vi "oa_TV Average Angle Intervals (1Chan).vi"(6 "revulotion index":i32, 7 "reset? (F)":bool, 8 "error in (no error)":errorcluster, 9 "pulse/revolution":i32, 10 "RPM":dbl[](array[numeric]), 11 "time index":dbl[](array[numeric]) format="%.2f") -> (0 "error out":errorcluster, 3 "angle intervals":dbl[](array[numeric]))   [LabVIEW 2017, in "SoundVib_Torsional.lvlib"]
uses:
  <vilib>/addons/Sound and Vibration/Order Analysis/Torsional Vibration/SoundVib_Torsional.lvlib
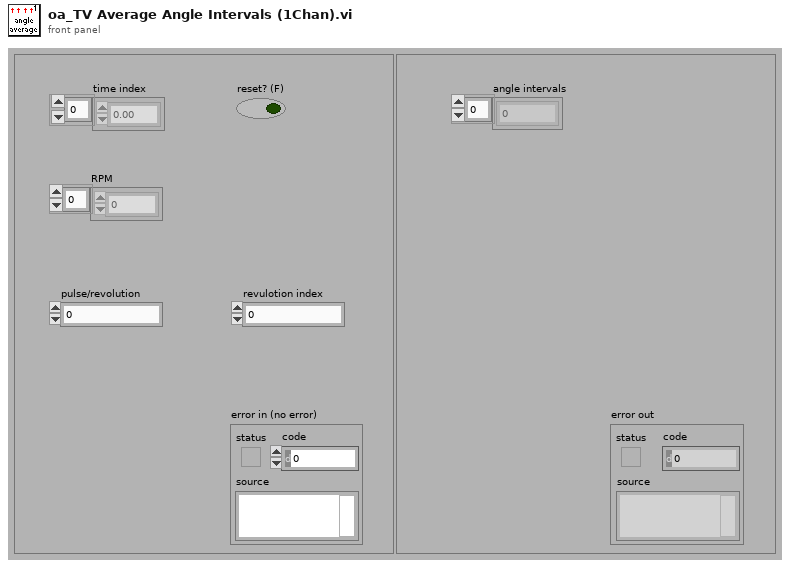
[diagram p1: front panel]
types:
  T1 = enum16{"Exponential average", "Moving average", "Current"}
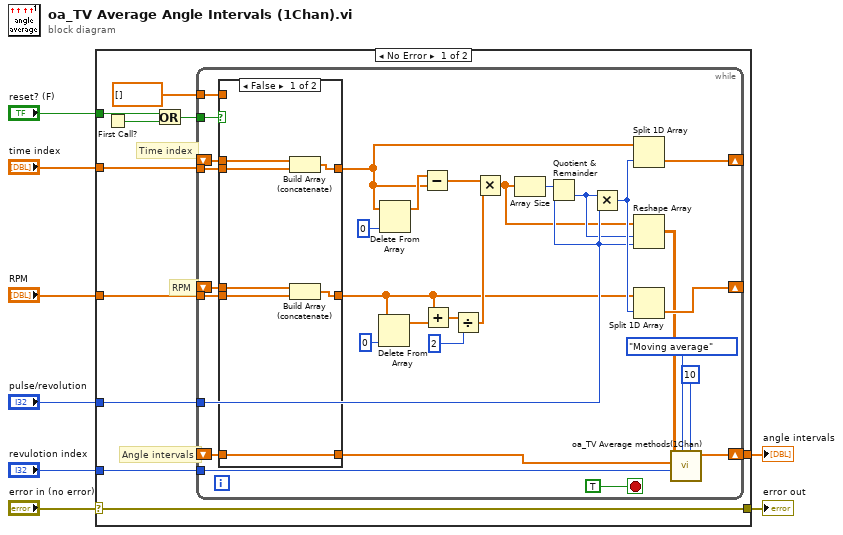
[diagram p0: block diagram]
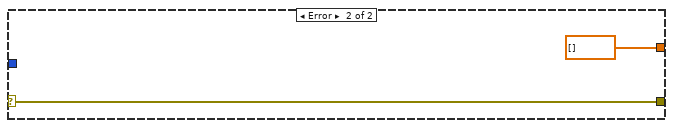
[diagram p3: hidden frame]
diagram:
  n1 = case shown="No Error" "error in (no error)" {
    selector: "error in (no error)" -> [w15 w60]
    tunnel: "time index" -> [w11 _]
    tunnel: "RPM" -> [w10 _]
    tunnel: "pulse/revolution" -> [w17 _]
    tunnel: "revulotion index" -> [w16 _]
    tunnel: [w14 dbl[] []] -> w4
    tunnel: [w15 w60] -> w2
    tunnel: "reset? (F)" -> [w9 _]
    frame No Error {
      # "Angle intervals"
      # "RPM"
      # "Time index"
      n2 = First Call?() -> (First Call?: T/F=w13:bool)
      n3 = Or(x=w9, y=w13) -> (x .or. y?=w12:bool)
      n4 = while {
        tunnel: w11 -> [w47]
        tunnel: w10 -> [w46]
        shift-right: [w36] -> _
        shift-left: _ -> [w49]
        shift-right: [w33] -> _
        shift-left: _ -> [w48]
        tunnel: w12 -> [w19]
        tunnel: dbl[] [] ("t") -> [w29]
        tunnel: w17 -> [w32]
        shift-right: [w24] -> w14
        shift-left: _ -> [w28]
        tunnel: w16 -> [w23]
        stop <- TRUE stop-if-true
        n5 = case shown="False" w19 {
          tunnel: w49 -> [w53 _]
          tunnel: w48 -> [w52 _]
          tunnel: w47 -> [w56 w59]
          tunnel: w46 -> [w55 w58]
          tunnel: [w54 w59] -> w37
          tunnel: w29 -> [_ w57]
          tunnel: w28 -> [w50 _]
          tunnel: [w51 w58] -> w27
          tunnel: [w50 w57] -> w25
          frame False {
            n6 = Build Array (concatenate)(w53, w56) -> (w54:dbl[])
            n7 = Build Array (concatenate)(w52, w55) -> (w51:dbl[])
          }
          frame True {
          }
        }
        n8 = Delete From Array(array=w27, index=0) -> (array with subset deleted=w38:dbl[])  [unwired: 1 in, 1 out]
        n9 = Delete From Array(array=w37, index=0) -> (array with subset deleted=w39:dbl[])  [unwired: 1 in, 1 out]
        n10 = Subtract(x=w39, y=w37) -> (x-y=w41:dbl[])
        n11 = Add(x=w27, y=w38) -> (x+y=w43:dbl[])
        n12 = Divide(x=w43, y=2) -> (x/y=w35:dbl[])
        n13 = Multiply(x=w41, y=w35) -> (x*y=w20:dbl[])
        n14 = Array Size(array=w20) -> (size(s)=w40:i32)
        n15 = Quotient & Remainder(x=w40, y=w32) -> (floor(x/y)=w31:i32)  [unwired: 1 out]
        n16 = Multiply(x=w31, y=w32) -> (x*y=w34:i32)
        n17 = Split 1D Array(array=w37, index=w34) -> (second subarray=w36:dbl[])  [unwired: 1 out]
        n18 = Reshape Array(w20, w31, w32) -> (w26:dbl[][])
        n19 = Split 1D Array(array=w27, index=w34) -> (second subarray=w33:dbl[])  [unwired: 1 out]
        n20 = call <vilib>:"oa_TV Average methods(1Chan).vi"("Window size"=i16 10, "Enum"=T1."Moving average", "Revulotion index"=w23, "Angle intervals"=w25, "Array"=w26) -> ("Angle intervals"=w24:dbl[])  [unwired: 6 in]
      }
    }
    frame Error {
    }
  }
  "error out" <- w2
  "angle intervals" <- w4
